vi "Inspect State Exec 1.vi"(8 "error in (no error)":errorcluster, 10 "Function":T31=enum."Exec", 11 "Image Src":T32) -> (0 "error out":errorcluster, 3 "Image Out":T32)   [LabVIEW 2019]
uses:
  <vilib>/vision/Image Controls.llb/IMAQ Image.ctl
  Common.llb/IVB Execution Function Code.ctl
  Common.llb/IVB Process Setup ROI.ctl
  Common.llb/IVB ROI Source.ctl
  IVB Simul IMAQ.llb/IVB Simul IMAQ - Parameters.ctl
  Common.llb/IVB String Result Value.ctl
  Common.llb/IVB Result Source.ctl
  Common.llb/IVB Measure ID.ctl
  Common.llb/IVB Calibration Data.ctl
  Common.llb/IVB Pass Fail Condition Array (Float).ctl
  Common.llb/IVB Pass Fail Condition (Float).ctl
  Common.llb/IVB Step Overlay Setup.ctl
  IVB VAA.llb/IVA VAA Lite Parameters.ctl
  IVB VAA.llb/IVA Script Step.ctl
  IVB Match Pattern.llb/IVB Match Pattern - Parameters.ctl
  IVB Match Pattern.llb/IVB Match Pattern - Sort Criteria.ctl
  IVB Match Geometric Pattern.llb/IVB Match Geometric Pattern - Parameters.ctl
  <vilib>/vision/Pattern Matching.llb/IMAQ Curve Parameters.ctl
  <vilib>/vision/Pattern Matching.llb/IMAQ Match Range Setting.ctl
  IVB Detect Objects.llb/IVB Detect Objects - Parameters.ctl
  Common.llb/IVB Threshold Data.ctl
  IVB Detect Objects.llb/IVB Detect Objects - Sorting Criteria.ctl
  Common.llb/IVB Particle Filter Data.ctl
  IVB OCR.llb/IVB OCR - Parameters.ctl
  IVB OCR.llb/IVB OCR - Pass Fail Condition.ctl
  Common.llb/IVB Pass Fail Condition (String).ctl
  IVB Overlay.llb/IVB Overlay - Parameters.ctl
  IVB Wait.llb/IVB Wait - Parameters.ctl
  Common.llb/IVB Numeric Result Value.ctl
  Common.llb/Inspect Script Step Subset.ctl
panel:
  in  "Overlay 8":T1=[TRUE, FALSE, FALSE, TRUE, FALSE, FALSE] caption="Overlay Setup 8"
  in  "Pass/Fail Condition 8":T2 {"Value 2" format="%.2f"; "Value 1" format="%.2f"}
  in  "Paramaters":T4={"Delay Type"=enum."Delay", "Time"={"Source"=enum."Constant", "Measure ID"={"Step GUID"="", "Result GUID"="", "Index"=0}, "Value"=1000.0}} caption="Parameters 8" {"Time"."Value" format="%.2f"}
  in  "ROI 8":T8 {"Constant ROI"."Contours"."Type" items=["No Selection", "Point", "Line", "Rectangle", "Oval", "Polygon", "Freehand Region", "Annulus", "Unused2", "Unused3", "Broken Line", "Freehand Line", "Rotated Rectangle"]}
  in  "Overlay 7":T1=[TRUE, FALSE, FALSE, TRUE, FALSE, FALSE] caption="Overlay Setup 7"
  in  "Pass/Fail Condition 7":T2 {"Value 2" format="%.2f"; "Value 1" format="%.2f"}
  in  "Parameters 6":T11={"Clear Previous Overlay"={"Source"=enum."Constant", "Measure ID"={"Step GUID"="", "Result GUID"="", "Index"=0}, "Value"=FALSE}, "Add Custom Overlay"={"Source"=enum."Constant", "Measure ID"={"Step GUID"="", "Result GUID"="", "Index"=0}, "Value"=TRUE}, "Custom Overlay"=[{"Name"="Rectangle 1", "Type"=enum."Rectangle", "Coordinates"=[{"Source"=enum."Constant", "Point ID"={"Step GUID"="", "Result GUID"="", "Index"=0}, "Coordinates"={"X"=211.0, "Y"=9.0}}, {"Source"=enum."Constant", "Point ID"={"Step GUID"="", "Result GUID"="", "Index"=0}, "Coordinates"={"X"=276.0, "Y"=39.0}}], "Dimensions"=[], "Results"=[], "Image File Path"=path "", "Use Keying Color"=FALSE, "Image GUID"="", "Text"="Your Text", "Colors"=[16711680, 16777216], "Font, Size & Style"={"Desired Font (Application)"=enum."User-specified Font", "[User-specified Font]"={"Font Name"="Tahoma", "Size"=13, "Strikeout?"=FALSE, "Italic?"=FALSE, "Underline?"=FALSE, "Outline?"=FALSE, "Shadow?"=FALSE, "Bold?"=TRUE, "Rotation Angle"=0.0}, "Horizontal Alignment"=0, "Vertical Alignment"=0}, "Width"=1}]} caption="Parameters 7" {"Custom Overlay"."Dimensions"."Value" format="%.2f"; "Custom Overlay"."Font, Size & Style"."Vertical Alignment" items=["Bottom", "Top", "Baseline"]; "Custom Overlay"."Font, Size & Style"."Horizontal Alignment" items=["Left", "Center", "Right"]; "Custom Overlay"."Font, Size & Style"."[User-specified Font]"."Rotation Angle" format="%.2f"; "Custom Overlay"."Coordinates"."Coordinates"."Y" format="%.2f"; "Custom Overlay"."Coordinates"."Coordinates"."X" format="%.2f"; "Custom Overlay"."Results"."Data Format" items=["String", "I8", "U8", "I16", "U16", "I32", "U32", "Single (4 bytes)", "Double (8 bytes)", "Extended (16 bytes)"]; "Custom Overlay"."Results"."Precision" min=0; "Custom Overlay"."Results"."Width" min=0; "Custom Overlay"."Results"."String Format" items=["Decimal", "Hexadecimal", "Octal", "Fractional", "Exponential", "Engineering"]}
  in  "ROI 7":T8 {"Constant ROI"."Contours"."Type" items=["No Selection", "Point", "Line", "Rectangle", "Oval", "Polygon", "Freehand Region", "Annulus", "Unused2", "Unused3", "Broken Line", "Freehand Line", "Rotated Rectangle"]}
  in  "Overlay 6":T1=[TRUE, FALSE, FALSE, TRUE, FALSE, FALSE] caption="Overlay Setup 6"
  in  "Pass/Fail Condition 6":T12={"Text Equal"={"Used"=FALSE, "Value 1"="", "Value 2"="", "Function"=enum."Equal"}, "Text Contains"={"Used"=FALSE, "Value 1"="", "Value 2"="", "Function"=enum."Match Pattern"}, "Identification Score"={"Used"=FALSE, "Value 1"=900.0, "Value 2"=0.0, "Function"=enum."Greater or Equal"}, "Confidence Score"={"Used"=FALSE, "Value 1"=900.0, "Value 2"=0.0, "Function"=enum."Greater or Equal"}} {"Confidence Score"."Value 2" format="%.2f"; "Confidence Score"."Value 1" format="%.2f"; "Identification Score"."Value 2" format="%.2f"; "Identification Score"."Value 1" format="%.2f"}
  in  "Parameters 5":T14={"Character Set Path"=path "G:/TRAIN LICENSE PLATE.abc", "Threshold Data"={"Method"=enum."Uniform", "Looking for"=1, "Color Mode"=0, "Kernel Size"={"Width"=32, "Height"=32}, "Ranges"=[{"Min"=1, "Max"=255}]}, "Reject Border"=TRUE, "Number Of Erosions"=0, "Number of Blocks"=4, "Size & Spacing"={"Segment Algorithm"=0, "Min Bounding Rect Width"=1, "Max Bounding Rect Width"=65536, "Min Bounding Rect Height"=1, "Max Bounding Rect Height"=65536, "Min Character Size"=20, "Max Character Size"=65536, "Min Char Spacing"=1, "Max Horiz Element Spacing"=1, "Max Vert Element Spacing"=0, "Min Space Distance"=65536}, "Read Options"={"Read Strategy"=1, "Read Resolution"=2, "Scale Dependant"=FALSE, "Aspect Ratio"=400, "Acceptance Level"=700, "Substitution Character"="?", "MultiLine"=TRUE}, "Valid Characters"=[], "Use Text Pattern"=FALSE, "Read or Verify"=enum."Read & Verify", "Exp. String"={"Source"=enum."Constant", "String ID"={"Step GUID"="", "Result GUID"="", "Index"=0}, "String"="?\r\n?\r\nIL?111AT"}, "Orientation"=0, "# Lines Expected"=0, "Internal File Name"="TRAIN LICENSE PLATE.abc"} caption="Parameters 6" {"Threshold Data"."Kernel Size"."Height" min=3; "Threshold Data"."Kernel Size"."Width" min=3; "Threshold Data"."Looking for" items=["Light on Dark", "Dark on Light"]; "Threshold Data"."Color Mode" items=["RGB", "HSL", "HSV", "HSI"]; "Orientation" items=["Baseline inside", "Baseline outside"]; "Valid Characters"."Pre-defined characters" items=["Any Character", "User-defined Characters", "Alphabetic", "Alphanumeric", "Uppercase Letters", "Lowercase Letters", "Decimal Digits", "Hexadecimal Digits", "Pattern", "Force Space"]; "Read Options"."Read Resolution" items=["Low", "Medium", "High"]; "Read Options"."Aspect Ratio" min=100; "Read Options"."Read Strategy" items=["Aggressive", "Conservative"]; "Read Options"."Acceptance Level" min=0 max=1000; "Size & Spacing"."Min Space Distance" min=0; "Size & Spacing"."Max Vert Element Spacing" min=0; "Size & Spacing"."Max Character Size" min=1; "Size & Spacing"."Max Horiz Element Spacing" min=1; "Size & Spacing"."Min Char Spacing" min=1; "Size & Spacing"."Segment Algorithm" items=["None", "Shortest Segment", "Legacy Auto Split"]; "Size & Spacing"."Min Bounding Rect Width" min=1; "Size & Spacing"."Min Character Size" min=1; "Size & Spacing"."Max Bounding Rect Height" min=1; "Size & Spacing"."Max Bounding Rect Width" min=1; "Size & Spacing"."Min Bounding Rect Height" min=1}
  in  "ROI 6":T8={"ROI Source"=enum."Constant", "Constant ROI"={"Global Rectangle"=[114, 219, 525, 489], "Contours"=[{"ID"=enum."External", "Type"=3, "Coordinates"=[114, 219, 525, 489]}]}, "Programmable ROI GUID"=""} {"Constant ROI"."Contours"."Type" items=["No Selection", "Point", "Line", "Rectangle", "Oval", "Polygon", "Freehand Region", "Annulus", "Unused2", "Unused3", "Broken Line", "Freehand Line", "Rotated Rectangle"]}
  in  "Overlay 5":T1=[TRUE, FALSE, FALSE, TRUE, FALSE, FALSE] caption="Overlay Setup 5"
  in  "Pass/Fail Condition 5":T2=[{"Used"=FALSE, "Value 1"=1.0, "Value 2"=0.0, "Function"=enum."Greater or Equal"}, {"Used"=FALSE, "Value 1"=1.0, "Value 2"=0.0, "Function"=enum."Less or Equal"}] {"Value 2" format="%.2f"; "Value 1" format="%.2f"}
  in  "Parameters 4":T15={"Threshold Settings"={"Image Type"=0, "Mono Data"={"Looking for"=1, "Method"=0, "AutoThresh Limits"={"Minimum"=10, "Maximum"=245}, "Kernel Size"={"Width"=35, "Height"=35}, "Deviation Factor"=0.2}, "Color Data"={"Color Mode"=1, "Exclude Hue Interval"=FALSE}, "Measurements"=[{"Source"=enum."Constant", "Measure ID"={"Step GUID"="", "Result GUID"="", "Index"=0}, "Value"=0.0}, {"Source"=enum."Constant", "Measure ID"={"Step GUID"="", "Result GUID"="", "Index"=0}, "Value"=128.0}, {"Source"=enum."Constant", "Measure ID"={"Step GUID"="", "Result GUID"="", "Index"=0}, "Value"=0.0}, {"Source"=enum."Constant", "Measure ID"={"Step GUID"="", "Result GUID"="", "Index"=0}, "Value"=255.0}, {"Source"=enum."Constant", "Measure ID"={"Step GUID"="", "Result GUID"="", "Index"=0}, "Value"=0.0}, {"Source"=enum."Constant", "Measure ID"={"Step GUID"="", "Result GUID"="", "Index"=0}, "Value"=255.0}]}, "Settings"={"Reject Border"=TRUE, "Fill Holes"=FALSE, "Min Object Size"=TRUE, "Min Size"=25.0, "Max Object Size"=TRUE, "Max Size"=1000.0}, "Sorting Criteria"=-1, "Order"=0, "Use Filter"=FALSE, "Filter Params"={"Filter Settings"=[], "Connectivity"=TRUE, "Remove"=FALSE}, "Object Params to Log"={"Pixel"=[0, 1, 35], "Real World"=[]}} caption="Parameters 5" {"Object Params to Log"."Real World" items=["Aspect Ratio"=-2, "Scan Order"=-1, "Center of Mass X"=0, "Center of Mass Y"=1, "First Pixel X"=2, "First Pixel Y"=3, "Bounding Rect Left"=4, "Bounding Rect Top"=5, "Bounding Rect Right"=6, "Bounding Rect Bottom"=7, "Max Feret Diameter Start X"=8, "Max Feret Diameter Start Y"=9, "Max Feret Diameter End X"=10, "Max Feret Diameter End Y"=11, "Max Horiz. Segment Length Left"=12, "Max Horiz. Segment Length Right"=13, "Max Horiz. Segment Length Row"=14, "-"=15, "Bounding Rect Width"=16, "Bounding Rect Height"=17, "Bounding Rect Diagonal"=18, "Perimeter"=19, "Convex Hull Perimeter"=20, "Holes' Perimeter"=21, "Max Feret Diameter"=22, "Equivalent Ellipse Major Axis"=23, "Equivalent Ellipse Minor Axis"=24, "Equivalent Ellipse Minor Axis (Feret)"=25, "Equivalent Rect Long Side"=26, "Equivalent Rect Short Side"=27, "Equivalent Rect Diagonal"=28, "Equivalent Rect Short Side (Feret)"=29, "Average Horiz. Segment Length"=30, "Average Vert. Segment Length"=31, "Hydraulic Radius"=32, "Waddel Disk Diameter"=33, "-"=34, "Area"=35, "Holes' Area"=36, "Particle & Holes' Area"=37, "Convex Hull Area"=38, "Image Area"=39, "-"=40, "Number of Holes"=41, "Number of Horiz. Segments"=42, "Number of Vert. Segments"=43, "-"=44, "Orientation"=45, "Max Feret Diameter Orientation"=46, "-"=47, "% Area/Image Area"=48, "% Area/(Particle & Holes' Area)"=49, "Ratio of Equivalent Ellipse Axes"=50, "Ratio of Equivalent Rect Sides"=51, "-"=52, "Elongation Factor"=53, "Compactness Factor"=54, "Heywood Circularity Factor"=55, "Type Factor"=56, "-"=57, "Sum X"=58, "Sum Y"=59, "Sum XX"=60, "Sum XY"=61, "Sum YY"=62, "Sum XXX"=63, "Sum XXY"=64, "Sum XYY"=65, "Sum YYY"=66, "-"=67, "Moment of Inertia XX"=68, "Moment of Inertia XY"=69, "Moment of Inertia YY"=70, "Moment of Inertia XXX"=71, "Moment of Inertia XXY"=72, "Moment of Inertia XYY"=73, "Moment of Inertia YYY"=74, "Norm. Moment of Inertia XX"=75, "Norm. Moment of Inertia XY"=76, "Norm. Moment of Inertia YY"=77, "Norm. Moment of Inertia XXX"=78, "Norm. Moment of Inertia XXY"=79, "Norm. Moment of Inertia XYY"=80, "Norm. Moment of Inertia YYY"=81, "Hu Moment 1"=82, "Hu Moment 2"=83, "Hu Moment 3"=84, "Hu Moment 4"=85, "Hu Moment 5"=86, "Hu Moment 6"=87, "Hu Moment 7"=88]; "Object Params to Log"."Pixel" items=["Aspect Ratio"=-2, "Scan Order"=-1, "Center of Mass X"=0, "Center of Mass Y"=1, "First Pixel X"=2, "First Pixel Y"=3, "Bounding Rect Left"=4, "Bounding Rect Top"=5, "Bounding Rect Right"=6, "Bounding Rect Bottom"=7, "Max Feret Diameter Start X"=8, "Max Feret Diameter Start Y"=9, "Max Feret Diameter End X"=10, "Max Feret Diameter End Y"=11, "Max Horiz. Segment Length Left"=12, "Max Horiz. Segment Length Right"=13, "Max Horiz. Segment Length Row"=14, "-"=15, "Bounding Rect Width"=16, "Bounding Rect Height"=17, "Bounding Rect Diagonal"=18, "Perimeter"=19, "Convex Hull Perimeter"=20, "Holes' Perimeter"=21, "Max Feret Diameter"=22, "Equivalent Ellipse Major Axis"=23, "Equivalent Ellipse Minor Axis"=24, "Equivalent Ellipse Minor Axis (Feret)"=25, "Equivalent Rect Long Side"=26, "Equivalent Rect Short Side"=27, "Equivalent Rect Diagonal"=28, "Equivalent Rect Short Side (Feret)"=29, "Average Horiz. Segment Length"=30, "Average Vert. Segment Length"=31, "Hydraulic Radius"=32, "Waddel Disk Diameter"=33, "-"=34, "Area"=35, "Holes' Area"=36, "Particle & Holes' Area"=37, "Convex Hull Area"=38, "Image Area"=39, "-"=40, "Number of Holes"=41, "Number of Horiz. Segments"=42, "Number of Vert. Segments"=43, "-"=44, "Orientation"=45, "Max Feret Diameter Orientation"=46, "-"=47, "% Area/Image Area"=48, "% Area/(Particle & Holes' Area)"=49, "Ratio of Equivalent Ellipse Axes"=50, "Ratio of Equivalent Rect Sides"=51, "-"=52, "Elongation Factor"=53, "Compactness Factor"=54, "Heywood Circularity Factor"=55, "Type Factor"=56, "-"=57, "Sum X"=58, "Sum Y"=59, "Sum XX"=60, "Sum XY"=61, "Sum YY"=62, "Sum XXX"=63, "Sum XXY"=64, "Sum XYY"=65, "Sum YYY"=66, "-"=67, "Moment of Inertia XX"=68, "Moment of Inertia XY"=69, "Moment of Inertia YY"=70, "Moment of Inertia XXX"=71, "Moment of Inertia XXY"=72, "Moment of Inertia XYY"=73, "Moment of Inertia YYY"=74, "Norm. Moment of Inertia XX"=75, "Norm. Moment of Inertia XY"=76, "Norm. Moment of Inertia YY"=77, "Norm. Moment of Inertia XXX"=78, "Norm. Moment of Inertia XXY"=79, "Norm. Moment of Inertia XYY"=80, "Norm. Moment of Inertia YYY"=81, "Hu Moment 1"=82, "Hu Moment 2"=83, "Hu Moment 3"=84, "Hu Moment 4"=85, "Hu Moment 5"=86, "Hu Moment 6"=87, "Hu Moment 7"=88]; "Sorting Criteria" items=["Aspect Ratio"=-2, "Scan Order"=-1, "Center of Mass X"=0, "Center of Mass Y"=1, "First Pixel X"=2, "First Pixel Y"=3, "Bounding Rect Left"=4, "Bounding Rect Top"=5, "Bounding Rect Right"=6, "Bounding Rect Bottom"=7, "Max Feret Diameter Start X"=8, "Max Feret Diameter Start Y"=9, "Max Feret Diameter End X"=10, "Max Feret Diameter End Y"=11, "Max Horiz. Segment Length Left"=12, "Max Horiz. Segment Length Right"=13, "Max Horiz. Segment Length Row"=14, "-"=15, "Bounding Rect Width"=16, "Bounding Rect Height"=17, "Bounding Rect Diagonal"=18, "Perimeter"=19, "Convex Hull Perimeter"=20, "Holes' Perimeter"=21, "Max Feret Diameter"=22, "Equivalent Ellipse Major Axis"=23, "Equivalent Ellipse Minor Axis"=24, "Equivalent Ellipse Minor Axis (Feret)"=25, "Equivalent Rect Long Side"=26, "Equivalent Rect Short Side"=27, "Equivalent Rect Diagonal"=28, "Equivalent Rect Short Side (Feret)"=29, "Average Horiz. Segment Length"=30, "Average Vert. Segment Length"=31, "Hydraulic Radius"=32, "Waddel Disk Diameter"=33, "-"=34, "Area"=35, "Holes' Area"=36, "Particle & Holes' Area"=37, "Convex Hull Area"=38, "Image Area"=39, "-"=40, "Number of Holes"=41, "Number of Horiz. Segments"=42, "Number of Vert. Segments"=43, "-"=44, "Orientation"=45, "Max Feret Diameter Orientation"=46, "-"=47, "% Area/Image Area"=48, "% Area/(Particle & Holes' Area)"=49, "Ratio of Equivalent Ellipse Axes"=50, "Ratio of Equivalent Rect Sides"=51, "-"=52, "Elongation Factor"=53, "Compactness Factor"=54, "Heywood Circularity Factor"=55, "Type Factor"=56, "-"=57, "Sum X"=58, "Sum Y"=59, "Sum XX"=60, "Sum XY"=61, "Sum YY"=62, "Sum XXX"=63, "Sum XXY"=64, "Sum XYY"=65, "Sum YYY"=66, "-"=67, "Moment of Inertia XX"=68, "Moment of Inertia XY"=69, "Moment of Inertia YY"=70, "Moment of Inertia XXX"=71, "Moment of Inertia XXY"=72, "Moment of Inertia XYY"=73, "Moment of Inertia YYY"=74, "Norm. Moment of Inertia XX"=75, "Norm. Moment of Inertia XY"=76, "Norm. Moment of Inertia YY"=77, "Norm. Moment of Inertia XXX"=78, "Norm. Moment of Inertia XXY"=79, "Norm. Moment of Inertia XYY"=80, "Norm. Moment of Inertia YYY"=81, "Hu Moment 1"=82, "Hu Moment 2"=83, "Hu Moment 3"=84, "Hu Moment 4"=85, "Hu Moment 5"=86, "Hu Moment 6"=87, "Hu Moment 7"=88]; "Settings"."Max Size" min=0.0 max=999999999.0 step=1.0 format="%.2f"; "Settings"."Min Size" min=0.0 max=999999999.0 step=1.0 format="%.2f"; "Threshold Settings"."Image Type" items=["Grayscale (U8)", "Grayscale (I16)", "Grayscale (SGL)", "Complex (CSG)", "RGB (U32)", "HSL (U32)", "RGB (U64)", "Grayscale (U16)"]; "Threshold Settings"."Measurements"."Value" format="%.2f"; "Threshold Settings"."Color Data"."Color Mode" items=["RGB", "HSL", "HSV", "HSI"]; "Threshold Settings"."Mono Data"."Deviation Factor" min=0.0 max=1.0 format="%.2f"; "Threshold Settings"."Mono Data"."Kernel Size"."Height" min=0 max=255 step=1; "Threshold Settings"."Mono Data"."Kernel Size"."Width" min=0 max=255 step=1; "Threshold Settings"."Mono Data"."AutoThresh Limits"."Maximum" min=0 max=255 step=1; "Threshold Settings"."Mono Data"."AutoThresh Limits"."Minimum" min=0 max=255 step=1; "Threshold Settings"."Mono Data"."Method" items=["Manual Threshold", "-", "Auto Threshold: Clustering", "Auto Threshold: Entropy", "Auto Threshold: Metric", "Auto Threshold: Moments", "Auto Threshold: Inter Variance", "-", "Local Threshold: Niblack", "Local Threshold: BG Correction"]; "Threshold Settings"."Mono Data"."Looking for" items=["Bright Objects", "Dark Objects", "Gray Objects"]; "Filter Params"."Filter Settings"."High"."Value" format="%.2f"; "Filter Params"."Filter Settings"."Low"."Value" format="%.2f"; "Filter Params"."Filter Settings"."Measurement" items=["Center of Mass X", "Center of Mass Y", "First Pixel X", "First Pixel Y", "Bounding Rect Left", "Bounding Rect Top", "Bounding Rect Right", "Bounding Rect Bottom", "Max Feret Diameter Start X", "Max Feret Diameter Start Y", "Max Feret Diameter End X", "Max Feret Diameter End Y", "Max Horiz. Segment Length Left", "Max Horiz. Segment Length Right", "Max Horiz. Segment Length Row", "-", "Bounding Rect Width", "Bounding Rect Height", "Bounding Rect Diagonal", "Perimeter", "Convex Hull Perimeter", "Holes' Perimeter", "Max Feret Diameter", "Equivalent Ellipse Major Axis", "Equivalent Ellipse Minor Axis", "Equivalent Ellipse Minor Axis (Feret)", "Equivalent Rect Long Side", "Equivalent Rect Short Side", "Equivalent Rect Diagonal", "Equivalent Rect Short Side (Feret)", "Average Horiz. Segment Length", "Average Vert. Segment Length", "Hydraulic Radius", "Waddel Disk Diameter", "-", "Area", "Holes' Area", "Particle & Holes' Area", "Convex Hull Area", "Image Area", "-", "Number of Holes", "Number of Horiz. Segments", "Number of Vert. Segments", "-", "Orientation", "Max Feret Diameter Orientation", "-", "% Area/Image Area", "% Area/(Particle & Holes' Area)", "Ratio of Equivalent Ellipse Axes", "Ratio of Equivalent Rect Sides", "-", "Elongation Factor", "Compactness Factor", "Heywood Circularity Factor", "Type Factor", "-", "Sum X", "Sum Y", "Sum XX", "Sum XY", "Sum YY", "Sum XXX", "Sum XXY", "Sum XYY", "Sum YYY", "-", "Moment of Inertia XX", "Moment of Inertia XY", "Moment of Inertia YY", "Moment of Inertia XXX", "Moment of Inertia XXY", "Moment of Inertia XYY", "Moment of Inertia YYY", "Norm. Moment of Inertia XX", "Norm. Moment of Inertia XY", "Norm. Moment of Inertia YY", "Norm. Moment of Inertia XXX", "Norm. Moment of Inertia XXY", "Norm. Moment of Inertia XYY", "Norm. Moment of Inertia YYY", "Hu Moment 1", "Hu Moment 2", "Hu Moment 3", "Hu Moment 4", "Hu Moment 5", "Hu Moment 6", "Hu Moment 7"]}
  in  "ROI 5":T8={"ROI Source"=enum."Constant", "Constant ROI"={"Global Rectangle"=[92, 229, 501, 509], "Contours"=[{"ID"=enum."External", "Type"=3, "Coordinates"=[92, 229, 501, 509]}]}, "Programmable ROI GUID"=""} {"Constant ROI"."Contours"."Type" items=["No Selection", "Point", "Line", "Rectangle", "Oval", "Polygon", "Freehand Region", "Annulus", "Unused2", "Unused3", "Broken Line", "Freehand Line", "Rotated Rectangle"]}
  in  "Overlay 4":T1=[TRUE, FALSE, FALSE, TRUE, FALSE, FALSE] caption="Overlay Setup 4"
  in  "Pass/Fail Condition 4":T2=[{"Used"=FALSE, "Value 1"=1.0, "Value 2"=0.0, "Function"=enum."Greater or Equal"}, {"Used"=FALSE, "Value 1"=1.0, "Value 2"=0.0, "Function"=enum."Less or Equal"}] {"Value 2" format="%.2f"; "Value 1" format="%.2f"}
  in  "Parameters 3":T21={"Options"={"Curve Parameters"={"Extraction Mode"=0, "Edge Threshold"=75, "Edge Filter Size"=1, "Min Length"=25, "Row Search Step Size"=15, "Col Search Step Size"=15, "Max Endpoint Gap"=10, "Closed"=FALSE, "Subpixel"=FALSE}, "Match Mode"={"Rotation"=TRUE, "Scale"=FALSE, "Occlusion"=FALSE, "Reserved"=FALSE, "Reserved"=FALSE, "Reserved"=FALSE}, "Range Settings"=[{"Match Constraints"=0, "Min"=0.0, "Max"=360.0}], "Number of Matches"=1, "Minimum Match Score"=800.0, "SubPixel Accuracy"=TRUE, "Advanced Geometric Match Options"=[], "Adv. Geometric Match Options 2"=[{"Setup Data Item"=22, "Item Value"=1.0}, {"Setup Data Item"=21, "Item Value"=0.0}, {"Setup Data Item"=15, "Item Value"=20.0}, {"Setup Data Item"=16, "Item Value"=10.0}, {"Setup Data Item"=17, "Item Value"=10.0}, {"Setup Data Item"=18, "Item Value"=80.0}, {"Setup Data Item"=14, "Item Value"=0.0}], "Sort Criteria"=enum."Score", "Sort Order"=enum."Descending"}, "Template Path"=path "C:/Users/Jerry/AppData/Local/Temp/VBAI/1932/93671840.png", "Algorithm"=enum."Geometric Matching"} caption="Parameters 4" {"Options"."Adv. Geometric Match Options 2"."Item Value" format="%.2f"; "Options"."Adv. Geometric Match Options 2"."Setup Data Item" items=["Curve Extraction Mode", "Curve Edge Threshold", "Curve Edge Filter Size", "Min Curve Length", "Curve Row Search Step Size", "Curve Col Search Step Size", "Curve Max Endpoint Gap", "Extract Closed Curves", "Enable Subpixel Curve Extraction", "Enable Correlation Score", "Enable Subpixel Accuracy", "Subpixel Iterations", "Subpixel Tolerance", "Initial Match List Length", "Enable Target Template Curve Score", "Min Match Separation Distance", "Min Match Separation Angle", "Min Match Separation Scale", "Max Match Overlap", "Enable Coarse Result", "Enable Calibration Support", "Enable Contrast Reversal", "Search Strategy", "Refinement Match Factor", "Subpixel Match Factor"]; "Options"."Advanced Geometric Match Options"."Item Value" format="%.2f"; "Options"."Advanced Geometric Match Options"."Setup Data Item" items=["Curve Extraction Mode", "Curve Edge Threshold", "Curve Edge Filter Size", "Min Curve Length", "Curve Row Search Step Size", "Curve Col Search Step Size", "Curve Max Endpoint Gap", "Extract Closed Curves", "Enable Subpixel Curve Extraction", "Min Features", "Max Features ", "Enable Correlation Score", "Enable Subpixel Accuracy", "Subpixel Iterations", "Subpixel Tolerance", "Initial Match List Length", "Enable Target Template Curve Score", "Min Match Separation Distance", "Min Match Separation Angle", "Min Match Separation Scale", "Max Match Overlap", "Enable Coarse Result"]; "Options"."Range Settings"."Match Constraints" items=["Rotation Angle (degrees)", "Scale Factor (%)", "Occlusion (%)"]; "Options"."Curve Parameters"."Max Endpoint Gap" min=0; "Options"."Curve Parameters"."Col Search Step Size" min=1 max=255 step=1; "Options"."Curve Parameters"."Row Search Step Size" min=1 max=255 step=1; "Options"."Curve Parameters"."Min Length" min=0; "Options"."Curve Parameters"."Edge Filter Size" items=["Fine", "Normal", "Controur Tracing"]; "Options"."Curve Parameters"."Edge Threshold" min=1 max=65535 step=1; "Options"."Curve Parameters"."Extraction Mode" items=["Normal", "Uniform Regions"]; "Options"."Minimum Match Score" min=0 max=1000 format="%.2f"; "Options"."Number of Matches" min=1}
  in  "ROI 4":T8={"ROI Source"=enum."Constant", "Constant ROI"={"Global Rectangle"=[0, 0, 640, 480], "Contours"=[{"ID"=enum."External", "Type"=3, "Coordinates"=[0, 0, 640, 480]}]}, "Programmable ROI GUID"=""} {"Constant ROI"."Contours"."Type" items=["No Selection", "Point", "Line", "Rectangle", "Oval", "Polygon", "Freehand Region", "Annulus", "Unused2", "Unused3", "Broken Line", "Freehand Line", "Rotated Rectangle"]}
  in  "Overlay 3":T1=[TRUE, FALSE, FALSE, TRUE, FALSE, FALSE] caption="Overlay Setup 3"
  in  "Pass/Fail Condition 3":T2=[{"Used"=FALSE, "Value 1"=1.0, "Value 2"=0.0, "Function"=enum."Greater or Equal"}, {"Used"=FALSE, "Value 1"=1.0, "Value 2"=0.0, "Function"=enum."Less or Equal"}] {"Value 2" format="%.2f"; "Value 1" format="%.2f"}
  in  "Parameters 2":T24={"Algorithm"=1, "# Matches"=1, "Min Match Score"=800.0, "Angle Ranges"=[], "Advanced Options"=[{"Item"=0, "Value"=10.0}, {"Item"=2, "Value"=2.0}, {"Item"=5, "Value"=300.0}, {"Item"=6, "Value"=3.0}, {"Item"=7, "Value"=5.0}, {"Item"=8, "Value"=2.0}, {"Item"=1, "Value"=1.0}, {"Item"=3, "Value"=20.0}, {"Item"=4, "Value"=0.0}], "Sort Criteria"=5, "Sort Order"=1} caption="Parameters 3" {"Advanced Options"."Item" items=["LD Sampling - Minimum Constrast"=0, "LD Sampling - Enable Subpixel Accuracy"=1, "LD Sampling - Search Strategy"=2, "LD Sampling - Subpixel Iterations"=3, "LD Sampling - Subpixel Tolerance"=4, "LD Sampling - Initial Match List Length"=5, "LD Sampling - Match List Reduction Factor"=6, "LD Sampling - Initial Step Size"=7, "LD Sampling - Intermediate Angular Accuracy"=8, "-"=9, "Pyramid - Max Pyramid Level"=100, "Pyramid - Minimum Contrast"=102, "Pyramid - Enable Subpixel Accuracy"=103, "Pyramid - Subpixel Iterations"=104, "Pyramid - Subpixel Tolerance"=105, "Pyramid - Initial Match List Length"=106, "Pyramid - Match List Reduction Factor"=107, "Pyramid - Intermediate Angular Accuracy"=108, "Pyramid - Process Border Matches"=109, "Pyramid - Min Match Separation Distance"=111, "Pyramid - Min Match Separation Angle"=112, "Pyramid - Max Match Overlap"=113, "Pyramid - Max Cache in MB"=114, "Pyramid - Clear Cache"=115]; "Algorithm" items=["All", "Low Discrepancy Sampling", "Grayscale Value Pyramid", "Gradients Pyramid"]; "Sort Order" items=["Ascending", "Descending"]; "Sort Criteria" items=["X Position (Pixels)", "Y Position (Pixels)", "X Position (Calibrated)", "Y Position (Calibrated)", "Angle (degrees)", "Score", "Angle (Calibrated)"]}
  in  "ROI 3":T8={"ROI Source"=enum."Full Image", "Constant ROI"={"Global Rectangle"=[0, 0, 640, 480], "Contours"=[{"ID"=enum."External", "Type"=3, "Coordinates"=[0, 0, 640, 480]}]}, "Programmable ROI GUID"=""} {"Constant ROI"."Contours"."Type" items=["No Selection", "Point", "Line", "Rectangle", "Oval", "Polygon", "Freehand Region", "Annulus", "Unused2", "Unused3", "Broken Line", "Freehand Line", "Rotated Rectangle"]}
  in  "Overlay 2":T1=[TRUE, FALSE, FALSE, TRUE, FALSE, FALSE] caption="Overlay Setup 2"
  in  "Pass/Fail Condition 2":T2 {"Value 2" format="%.2f"; "Value 1" format="%.2f"}
  in  "VAA Lite Parameters":T26=[{"Step Path"=path "C:/Program Files (x86)/National Instruments/Vision Builder AI 2015/VAA/Plugins/22 IVA CLRThreshold.llb/IVA CLRThreshold Exec.vi", "Step Setup"={"Process"="Color Threshold", "Name"="Color Threshold 1", "Process ID"="13591135", "Reference"="", "Ref Position"="", "Init Setup"=variant, "Setup"=variant(cluster{"Color Model":u16, "RHH Range":cluster{"Lower value":u8, "Upper value":u8}, "GSS Range":cluster{"Lower value":u8, "Upper value":u8}, "BLV Range":cluster{"Lower value":u8, "Upper value":u8}, "In / Out":bool} {"Color Model"=0, "RHH Range"={"Lower value"=64, "Upper value"=255}, "GSS Range"={"Lower value"=59, "Upper value"=233}, "BLV Range"={"Lower value"=50, "Upper value"=255}, "In / Out"=FALSE}), "PF Criteria"=variant, "Overlay"=[TRUE, FALSE, FALSE, TRUE, FALSE, FALSE], "Palette"="Binary", "(Reserved)"="IMAQ ColorThreshold"}}, {"Step Path"=path "C:/Program Files (x86)/National Instruments/Vision Builder AI 2015/VAA/Plugins/30 IVA GrayLookup.llb/IVA GrayLookup Exec.vi", "Step Setup"={"Process"="Lookup Table", "Name"="Lookup Table 1", "Process ID"="13594157", "Reference"="", "Ref Position"="", "Init Setup"=variant, "Setup"=variant(cluster{"Operator":u32, "Power Value":sgl, "Process":i32} {"Operator"=0, "Power Value"=1.0, "Process"=2}), "PF Criteria"=variant, "Overlay"=[TRUE, TRUE, TRUE, TRUE, TRUE, FALSE], "Palette"="Grayscale", "(Reserved)"="IMAQ Equalize"}}] caption="Parameters 2"
  in  "ROI 2":T8={"ROI Source"=enum."Full Image", "Constant ROI"={"Global Rectangle"=[0, 0, 640, 480], "Contours"=[{"ID"=enum."External", "Type"=3, "Coordinates"=[0, 0, 640, 480]}]}, "Programmable ROI GUID"=""} {"Constant ROI"."Contours"."Type" items=["No Selection", "Point", "Line", "Rectangle", "Oval", "Polygon", "Freehand Region", "Annulus", "Unused2", "Unused3", "Broken Line", "Freehand Line", "Rotated Rectangle"]}
  in  "Overlay":T1=[TRUE, FALSE, FALSE, TRUE, FALSE, FALSE] caption="Overlay Setup 1"
  in  "Pass/Fail Condition":T2 caption="Pass/Fail Condition 1" {"Value 2" format="%.2f"; "Value 1" format="%.2f"}
  in  "Parameters":T28={"Path"={"Source"=enum."Constant", "Measure ID"={"Step GUID"="", "Result GUID"="", "Index"=0}, "Value"="F:\\¬R¥ô\\picture\\P1010001.jpg"}, "Cycle through images"=TRUE, "Cache Images"=FALSE, "Calibration Data"={"Calibrate"=FALSE, "Calibration Name"="", "Correct Image"=FALSE, "Correction Data"={"Interpolation Type"=0, "Replace Value"=0.0}}, "Read Extra Info"=FALSE, "Set Bit Depth"=FALSE, "Bit Depth"=10} caption="Parameters 1" {"Calibration Data"."Correction Data"."Interpolation Type" items=["Zero Order", "Bi-linear"]}
  in  "ROI":T8 caption="ROI 1" {"Constant ROI"."Contours"."Type" items=["No Selection", "Point", "Line", "Rectangle", "Oval", "Polygon", "Freehand Region", "Annulus", "Unused2", "Unused3", "Broken Line", "Freehand Line", "Rotated Rectangle"]}
  # "Simulate Acquisition 1"
  # "Vision Assistant 1"
  # "Match Pattern 1"
  # "Geometric Matching 1"
  # "Detect Objects 1"
  # "Read/Verify Text 1"
  # "Custom Overlay 1"
  # "Delay 1"
  # "Range"
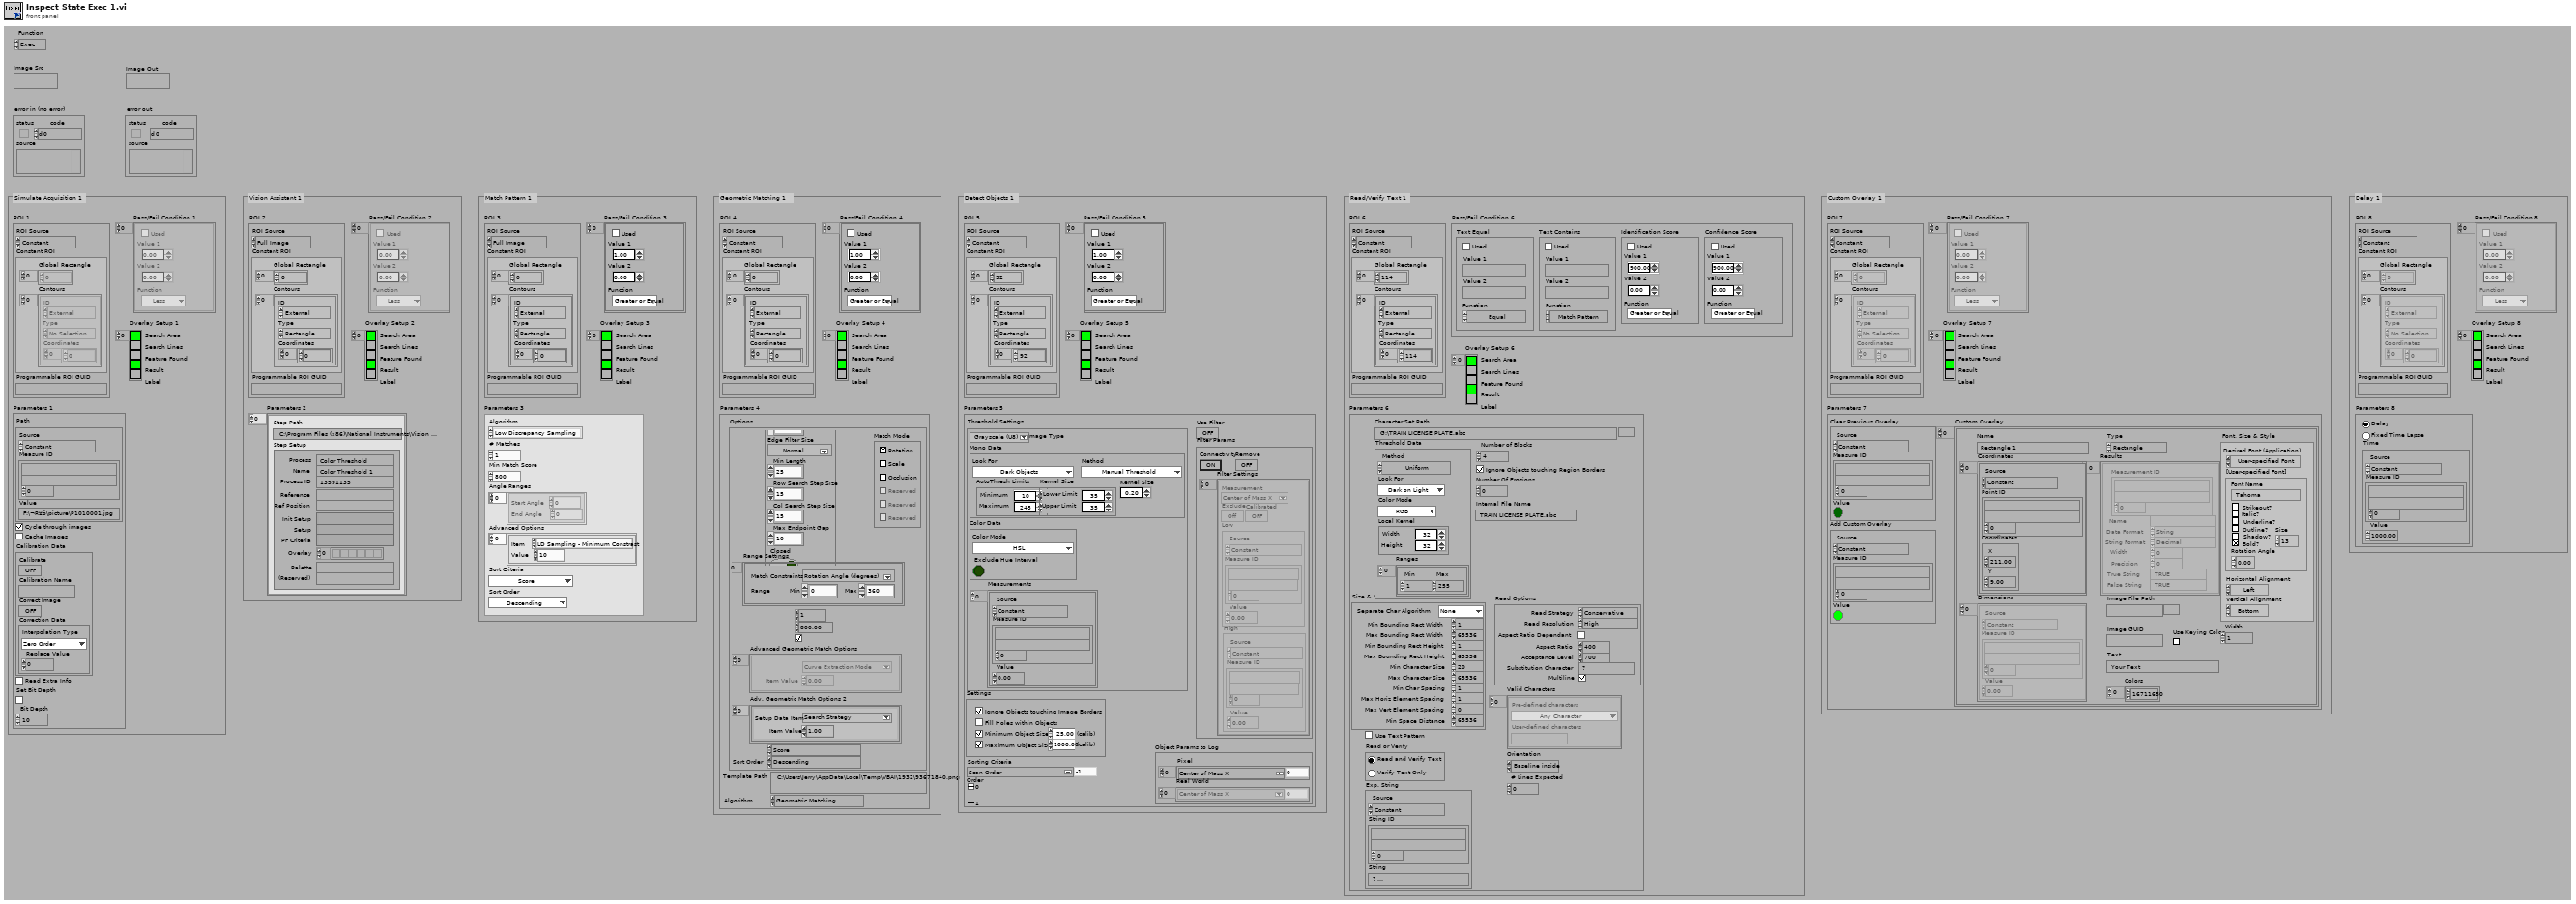
[diagram p1: front panel]
types:
  T1 = typedef "IVB Step Overlay Setup.ctl" = bool[]
  T2 = typedef "IVB Pass Fail Condition Array (Float).ctl" = T3[]
  T3 = typedef "IVB Pass Fail Condition (Float).ctl" = cluster{"Used":bool, "Value 1":dbl, "Value 2":dbl, "Function":enum16{"Less", "Less or Equal", "Greater", "Greater or Equal", "In Range", "Equal", "Not Equal"}}
  T4 = typedef "IVB Wait - Parameters.ctl" = cluster{"Delay Type":enum32{"Delay", "Time Lapse"}, "Time":T5}
  T5 = typedef "IVB Numeric Result Value.ctl" = cluster{"Source":T6, "Measure ID":T7, "Value":dbl}
  T6 = typedef "IVB Result Source.ctl" = enum16{"Constant", "Measure"}
  T7 = typedef "IVB Measure ID.ctl" = cluster{"Step GUID":string, "Result GUID":string, "Index":i32}
  T8 = typedef "IVB Process Setup ROI.ctl" = cluster{"ROI Source":T9, "Constant ROI":T10, "Programmable ROI GUID":string}
  T9 = typedef "IVB ROI Source.ctl" = enum16{"Constant", "Programmable", "Full Image"}
  T10 = typedef "ROI Descriptor" = cluster{"Global Rectangle":i32[], "Contours":cluster{"ID":enum32{"External", "Internal"}, "Type":u32, "Coordinates":i32[]}[]}
  T11 = typedef "IVB Overlay - Parameters.ctl" = cluster{"Clear Previous Overlay":cluster{"Source":enum16{"Constant", "Measure"}, "Measure ID":cluster{"Step GUID":string, "Result GUID":string, "Index":i32}, "Value":bool}, "Add Custom Overlay":cluster{"Source":enum16{"Constant", "Measure"}, "Measure ID":cluster{"Step GUID":string, "Result GUID":string, "Index":i32}, "Value":bool}, "Custom Overlay":cluster{"Name":string, "Type":enum16{"Point", "Line", "Rectangle", "Rotated Rectangle", "Oval", "Boolean Indicator", "Bitmap", "Text"}, "Coordinates":cluster{"Source":enum16{"Constant", "Measure"}, "Point ID":cluster{"Step GUID":string, "Result GUID":string, "Index":i32}, "Coordinates":cluster{"X":dbl, "Y":dbl}}[], "Dimensions":cluster{"Source":enum16{"Constant", "Measure"}, "Measure ID":cluster{"Step GUID":string, "Result GUID":string, "Index":i32}, "Value":dbl}[], "Results":cluster{"Measurement ID":cluster{"Step GUID":string, "Result GUID":string, "Index":i32}, "Name":string, "Data Format":u16, "String Format":u16, "Width":i16, "Precision":i16, "True String":string, "False String":string}[], "Image File Path":path, "Use Keying Color":bool, "Image GUID":string, "Text":string, "Colors":u32[], "Font, Size & Style":cluster{"Desired Font (Application)":enum16{"User-specified Font", "Application Font", "System Font", "Dialog Font"}, "[User-specified Font]":cluster{"Font Name":string, "Size":i16, "Strikeout?":bool, "Italic?":bool, "Underline?":bool, "Outline?":bool, "Shadow?":bool, "Bold?":bool, "Rotation Angle":dbl}, "Horizontal Alignment":i16, "Vertical Alignment":i16}, "Width":u32}[]}
  T12 = typedef "IVB OCR - Pass Fail Condition.ctl" = cluster{"Text Equal":T13, "Text Contains":T13, "Identification Score":T3, "Confidence Score":T3}
  T13 = typedef "IVB Pass Fail Condition (String).ctl" = cluster{"Used":bool, "Value 1":string, "Value 2":string, "Function":enum16{"Equal", "Not equal", "Match Pattern", "Less", "Less or Equal", "Greater", "Greater or Equal", "In Range"}}
  T14 = typedef "IVB OCR - Parameters.ctl" = cluster{"Character Set Path":path, "Threshold Data":cluster{"Method":enum16{"Fixed Range", "Uniform", "Linear", "Non Linear", "Local", "Color"}, "Looking for":u32, "Color Mode":u32, "Kernel Size":cluster{"Width":i32, "Height":i32}, "Ranges":cluster{"Min":i32, "Max":i32}[]}, "Reject Border":bool, "Number Of Erosions":i32, "Number of Blocks":i32, "Size & Spacing":cluster{"Segment Algorithm":u16, "Min Bounding Rect Width":i32, "Max Bounding Rect Width":i32, "Min Bounding Rect Height":i32, "Max Bounding Rect Height":i32, "Min Character Size":i32, "Max Character Size":i32, "Min Char Spacing":i32, "Max Horiz Element Spacing":i32, "Max Vert Element Spacing":i32, "Min Space Distance":i32}, "Read Options":cluster{"Read Strategy":i32, "Read Resolution":i32, "Scale Dependant":bool, "Aspect Ratio":i32, "Acceptance Level":i32, "Substitution Character":string, "MultiLine":bool}, "Valid Characters":cluster{"Pre-defined characters":i32, "User-defined characters":string}[], "Use Text Pattern":bool, "Read or Verify":enum32{"Read & Verify", "Verify Only"}, "Exp. String":cluster{"Source":enum16{"Constant", "Measure"}, "String ID":T7, "String":string}, "Orientation":u32, "# Lines Expected":u32, "Internal File Name":string}
  T15 = typedef "IVB Detect Objects - Parameters.ctl" = cluster{"Threshold Settings":T16, "Settings":cluster{"Reject Border":bool, "Fill Holes":bool, "Min Object Size":bool, "Min Size":dbl, "Max Object Size":bool, "Max Size":dbl}, "Sorting Criteria":T18, "Order":u32, "Use Filter":bool, "Filter Params":T19, "Object Params to Log":cluster{"Pixel":T18[], "Real World":T18[]}}
  T16 = typedef "IVB Threshold Data.ctl" = cluster{"Image Type":T17, "Mono Data":cluster{"Looking for":u32, "Method":u32, "AutoThresh Limits":cluster{"Minimum":i32, "Maximum":i32}, "Kernel Size":cluster{"Width":i32, "Height":i32}, "Deviation Factor":dbl}, "Color Data":cluster{"Color Mode":u32, "Exclude Hue Interval":bool}, "Measurements":cluster{"Source":enum16{"Constant", "Measure"}, "Measure ID":T7, "Value":dbl}[]}
  T17 = typedef "Image Type" = u32
  T18 = typedef "IVB Detect Objects - Sorting Criteria.ctl" = i32
  T19 = typedef "IVB Particle Filter Data.ctl" = cluster{"Filter Settings":cluster{"Measurement":T20, "Exclude":bool, "Calibrated":bool, "Low":cluster{"Source":T6, "Measure ID":T7, "Value":dbl}, "High":cluster{"Source":T6, "Measure ID":T7, "Value":dbl}}[], "Connectivity":bool, "Remove":bool}
  T20 = typedef "Particle Parameters" = i32
  T21 = typedef "IVB Match Geometric Pattern - Parameters.ctl" = cluster{"Options":cluster{"Curve Parameters":T22, "Match Mode":cluster{"Rotation":bool, "Scale":bool, "Occlusion":bool, "Reserved":bool, "Reserved":bool, "Reserved":bool}, "Range Settings":T23[], "Number of Matches":i32, "Minimum Match Score":sgl, "SubPixel Accuracy":bool, "Advanced Geometric Match Options":cluster{"Setup Data Item":u16, "Item Value":dbl}[], "Adv. Geometric Match Options 2":cluster{"Setup Data Item":u16, "Item Value":dbl}[], "Sort Criteria":enum16{"Score", "X Position (Pixels)", "Y Position (Pixels)", "X Position (Real World)", "Y Position (Real World)", "Angle", "Scale", "Occlusion %", "Template Target Curve Score", "Correlation Score", "Target Template Curve Score"}, "Sort Order":enum16{"Ascending", "Descending"}}, "Template Path":path, "Algorithm":enum32{"Geometric Matching", "Geometric Matching (Legacy)"}}
  T22 = typedef "IMAQ Curve Parameters.ctl" = cluster{"Extraction Mode":u32, "Edge Threshold":i32, "Edge Filter Size":u32, "Min Length":i32, "Row Search Step Size":i32, "Col Search Step Size":i32, "Max Endpoint Gap":i32, "Closed":bool, "Subpixel":bool}
  T23 = typedef "IMAQ Match Range Setting.ctl" = cluster{"Match Constraints":u32, "Min":dbl, "Max":dbl}
  T24 = typedef "IVB Match Pattern - Parameters.ctl" = cluster{"Algorithm":i32, "# Matches":i32, "Min Match Score":sgl, "Angle Ranges":cluster{"Start Angle":sgl, "End Angle":sgl}[], "Advanced Options":cluster{"Item":u16, "Value":dbl}[], "Sort Criteria":T25, "Sort Order":u32}
  T25 = typedef "IVB Match Pattern - Sort Criteria.ctl" = u32
  T26 = typedef "IVA VAA Lite Parameters.ctl" = cluster{"Step Path":path, "Step Setup":T27}[]
  T27 = typedef "IVA Script Step.ctl" = cluster{"Process":string, "Name":string, "Process ID":string, "Reference":string, "Ref Position":string, "Init Setup":variant, "Setup":variant, "PF Criteria":variant, "Overlay":bool[], "Palette":string, "(Reserved)":string}
  T28 = typedef "IVB Simul IMAQ - Parameters.ctl" = cluster{"Path":T29, "Cycle through images":bool, "Cache Images":bool, "Calibration Data":T30, "Read Extra Info":bool, "Set Bit Depth":bool, "Bit Depth":i32}
  T29 = typedef "IVB String Result Value.ctl" = cluster{"Source":T6, "Measure ID":T7, "Value":string}
  T30 = typedef "IVB Calibration Data.ctl" = cluster{"Calibrate":bool, "Calibration Name":string, "Correct Image":bool, "Correction Data":cluster{"Interpolation Type":u16, "Replace Value":sgl}}
  T31 = typedef "IVB Execution Function Code.ctl" = enum16{"Setup", "Exec", "Cleanup"}
  T32 = typedef "IMAQ Image.ctl" = refnum<image>
  T33 = typedef "Inspect Script Step Subset.ctl" = cluster{"GUID":string, "Name":string, "Process Class":string, "Disable":bool, "Reference ID":string, "Ref Position":string, "Palette":string}
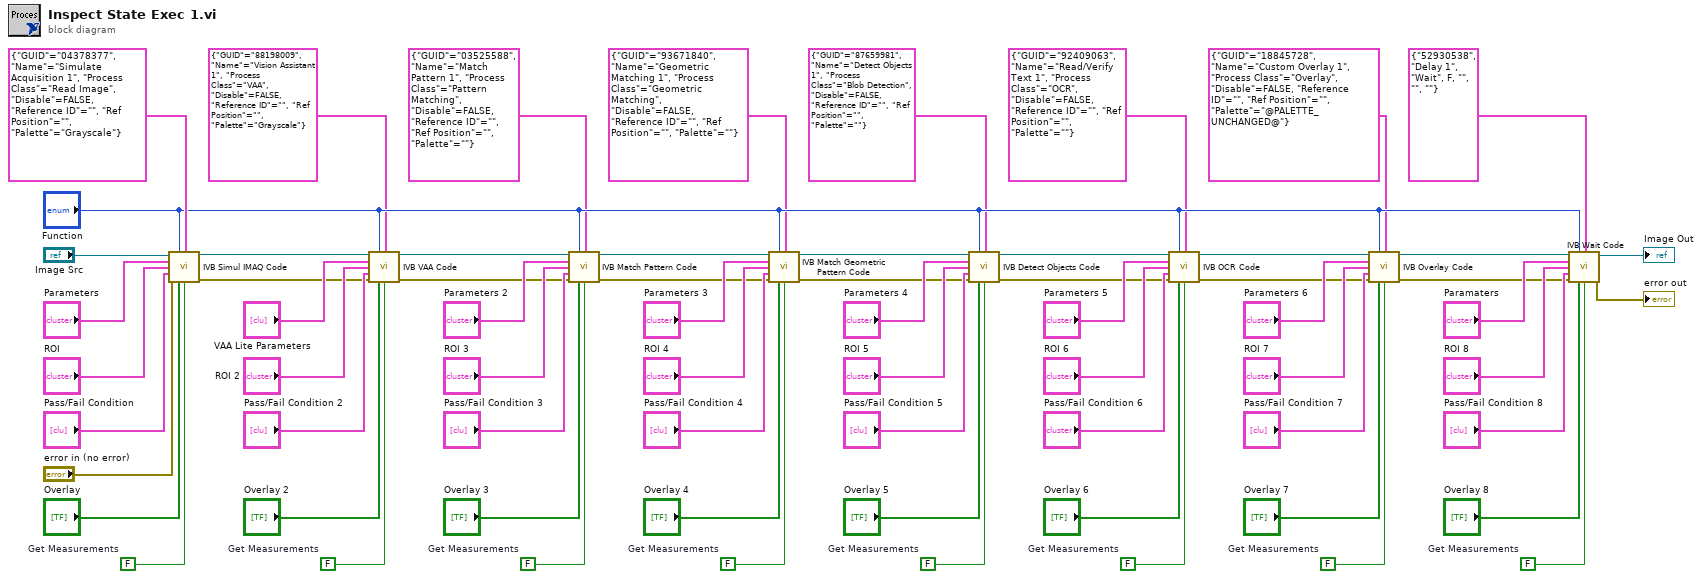
[diagram p0: block diagram]
diagram:
  w19 = FALSE  # Get Measurements
  w25 = FALSE  # Get Measurements
  w31 = FALSE  # Get Measurements
  w37 = FALSE  # Get Measurements
  w43 = FALSE  # Get Measurements
  w49 = FALSE  # Get Measurements
  w55 = FALSE  # Get Measurements
  w61 = FALSE  # Get Measurements
  n1 = call "IVB Simul IMAQ Code.vi"("Image Src"="Image Src", "Function"="Function", "Common Parameters"=T33 {"GUID"="04378377", "Name"="Simulate Acquisition 1", "Process Class"="Read Image", "Disable"=FALSE, "Reference ID"="", "Ref Position"="", "Palette"="Grayscale"}, "Parameters"="Parameters", "ROI"="ROI", "Pass/Fail Condition"="Pass/Fail Condition", "error in (no error)"="error in (no error)", "Overlay"="Overlay", "Get Measurements"=w61) -> ("Image Out"=w18:T32, "error out"=w17:errorcluster)  [unwired: 4 in, 1 out]
  n2 = call "IVB VAA Code.vi"("Image Src"=w18, "Function"="Function", "Common Parameters"=T33 {"GUID"="88198009", "Name"="Vision Assistant 1", "Process Class"="VAA", "Disable"=FALSE, "Reference ID"="", "Ref Position"="", "Palette"="Grayscale"}, "Parameters"="VAA Lite Parameters", "ROI"="ROI 2", "Pass/Fail Condition"="Pass/Fail Condition 2", "error in (no error)"=w17, "Overlay"="Overlay 2", "Get Measurements"=w55) -> ("Image Out"=w16:T32, "error out"=w15:errorcluster)  [unwired: 4 in, 1 out]
  n3 = call "IVB Match Pattern Code.vi"("Image Src"=w16, "Function"="Function", "Common Parameters"=T33 {"GUID"="03525588", "Name"="Match Pattern 1", "Process Class"="Pattern Matching", "Disable"=FALSE, "Reference ID"="", "Ref Position"="", "Palette"=""}, "Parameters"="Parameters 2", "ROI"="ROI 3", "Pass/Fail Condition"="Pass/Fail Condition 3", "error in (no error)"=w15, "Overlay"="Overlay 3", "Get Measurements"=w49) -> ("Image Out"=w14:T32, "error out"=w13:errorcluster)  [unwired: 4 in, 1 out]
  n4 = call "IVB Match Geometric Pattern Code.vi"("Image Src"=w14, "Function"="Function", "Common Parameters"=T33 {"GUID"="93671840", "Name"="Geometric Matching 1", "Process Class"="Geometric Matching", "Disable"=FALSE, "Reference ID"="", "Ref Position"="", "Palette"=""}, "Parameters"="Parameters 3", "ROI"="ROI 4", "Pass/Fail Condition"="Pass/Fail Condition 4", "error in (no error)"=w13, "Overlay"="Overlay 4", "Get Measurements"=w43) -> ("Image Out"=w12:T32, "error out"=w11:errorcluster)  [unwired: 4 in, 1 out]
  n5 = call "IVB Detect Objects Code.vi"("Image Src"=w12, "Function"="Function", "Common Parameters"=T33 {"GUID"="87659981", "Name"="Detect Objects 1", "Process Class"="Blob Detection", "Disable"=FALSE, "Reference ID"="", "Ref Position"="", "Palette"=""}, "Parameters"="Parameters 4", "ROI"="ROI 5", "Pass/Fail Condition"="Pass/Fail Condition 5", "error in (no error)"=w11, "Overlay"="Overlay 5", "Get Measurements"=w37) -> ("Image Out"=w10:T32, "error out"=w9:errorcluster)  [unwired: 4 in, 1 out]
  n6 = call "IVB OCR Code.vi"("Image Src"=w10, "Function"="Function", "Common Parameters"=T33 {"GUID"="92409063", "Name"="Read/Verify Text 1", "Process Class"="OCR", "Disable"=FALSE, "Reference ID"="", "Ref Position"="", "Palette"=""}, "Parameters"="Parameters 5", "ROI"="ROI 6", "Pass/Fail Condition"="Pass/Fail Condition 6", "error in (no error)"=w9, "Overlay"="Overlay 6", "Get Measurements"=w31) -> ("Image Out"=w8:T32, "error out"=w7:errorcluster)  [unwired: 4 in, 1 out]
  n7 = call "IVB Overlay Code.vi"("Image Src"=w8, "Function"="Function", "Common Parameters"=T33 {"GUID"="18845728", "Name"="Custom Overlay 1", "Process Class"="Overlay", "Disable"=FALSE, "Reference ID"="", "Ref Position"="", "Palette"="@PALETTE_UNCHANGED@"}, "Parameters"="Parameters 6", "ROI"="ROI 7", "Pass/Fail Condition"="Pass/Fail Condition 7", "error in (no error)"=w7, "Overlay"="Overlay 7", "Get Measurements"=w25) -> ("Image Out"=w6:T32, "error out"=w5:errorcluster)  [unwired: 4 in, 1 out]
  n8 = call "IVB Wait Code.vi"("Image Src"=w6, "Function"="Function", "Common Parameters"=T33 {"GUID"="52930538", "Name"="Delay 1", "Process Class"="Wait", "Disable"=FALSE, "Reference ID"="", "Ref Position"="", "Palette"=""}, "Parameters"="Paramaters", "ROI"="ROI 8", "Pass/Fail Condition"="Pass/Fail Condition 8", "error in (no error)"=w5, "Overlay"="Overlay 8", "Get Measurements"=w19) -> ("Image Out"=→"Image Out":T32, "error out"=→"error out":errorcluster)  [unwired: 4 in, 1 out]
